vi "LsitBox Add.vi"() -> ()   [LabVIEW 2011]
panel:
  in  "stop":bool
  out "Selected":i32(listbox)
  in  "Delete":bool
  in  "Add":bool
  in  "Action":i32(listbox)
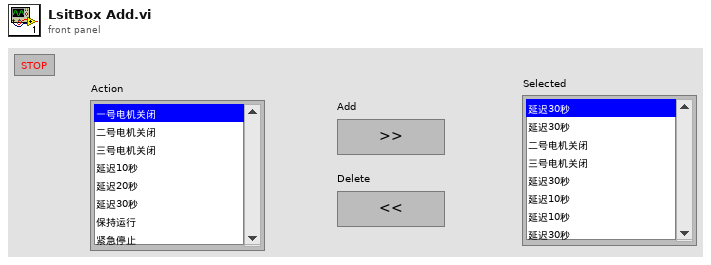
[diagram p1: front panel]
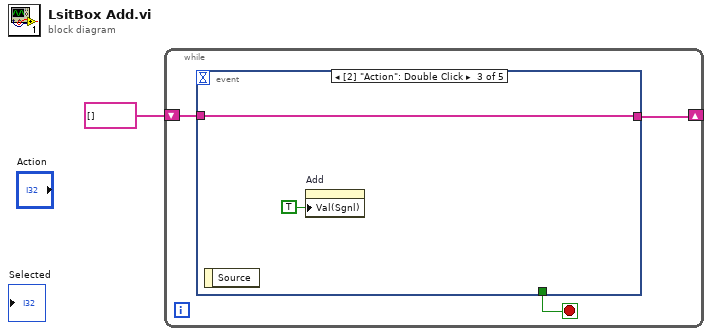
[diagram p0: block diagram]
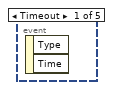
[diagram p2: hidden frame]
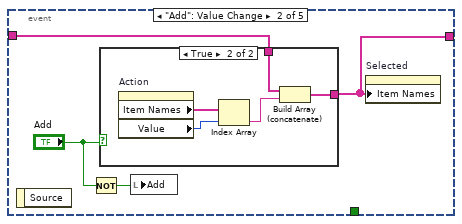
[diagram p3: hidden frame]
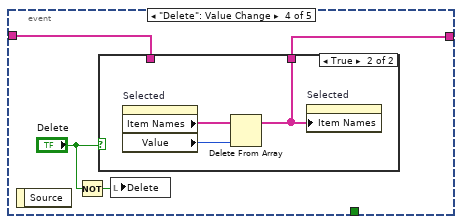
[diagram p5: hidden frame]
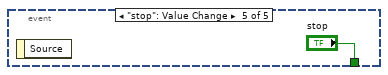
[diagram p7: hidden frame]
diagram:
  n1 = while {
    shift-right: [w2] -> _
    shift-left: string[] [] -> [w4]
    stop <- w3 stop-if-true
    n2 = event shown="[2] \"Action\": Double Click" {
      selector: _ -> [_ _ _ _ _]
      dyn-events: _ -> [_ _ _ _ _]
      timeout: _ -> [_ _ _ _ _]
      tunnel: w4 -> [_ w6 w16 w20 _]
      tunnel: [_ _ _ _ "stop"] -> w3
      tunnel: [_ w5 w16 w19 _] -> w2
      event Timeout {
        n3 = event-data() -> ()  [unwired: 1 in, 2 out]
      }
      event "Add": Value Change {
        n4 = event-data() -> ()  [unwired: 1 in, 1 out]
        n5 = Not(x="Add") -> (.not. x?=w8:bool)
        n6 = case shown="True" "Add" {
          tunnel: w6 -> [w9 w12]
          tunnel: [w9 w10] -> w5
          frame False {
          }
          frame True {
            n7 = property on="Action" class="LstBox (strict)"() -> ("Item Names"=w14:string[], "Value"=w13:i32)  [unwired: 2 in, 2 out]
            n8 = Index Array(array=w14, index=w13) -> (element=w11:string)
            n9 = Build Array (concatenate)(w12, w11) -> (w10:string[])
          }
        }
        n10 = local write "Add"(w8) -> ()
        n11 = property on="Selected" class="LstBox (strict)"("Item Names"=w5) -> ()  [unwired: 2 in, 2 out]
      }
      event "Action": Double Click {
        n12 = event-data() -> ()  [unwired: 1 in, 1 out]
        n13 = property on="Add" class="Bool (strict)"("Val(Sgnl)"=TRUE ("Value (Signaling)")) -> ()  [unwired: 2 in, 2 out]
      }
      event "Delete": Value Change {
        n14 = event-data() -> ()  [unwired: 1 in, 1 out]
        n15 = Not(x="Delete") -> (.not. x?=w18:bool)
        n16 = case shown="True" "Delete" {
          tunnel: w20 -> [w21 _]
          tunnel: [w21 w22] -> w19
          frame False {
          }
          frame True {
            n17 = property on="Selected" class="LstBox (strict)"() -> ("Item Names"=w23:string[], "Value"=w24:i32)  [unwired: 2 in, 2 out]
            n18 = Delete From Array(array=w23, index=w24) -> (array with subset deleted=w22:string[])  [unwired: 1 in, 1 out]
            n19 = property on="Selected" class="LstBox (strict)"("Item Names"=w22) -> ()  [unwired: 2 in, 2 out]
          }
        }
        n20 = local write "Delete"(w18) -> ()
      }
      event "stop": Value Change {
        n21 = event-data() -> ()  [unwired: 1 in, 1 out]
      }
    }
  }
